vi "GetDesiredHeading.vi"(10 "QueueRef":T1, 11 "NotifierReff":T2) -> (3 "Desired Heading":dbl)   [LabVIEW 2013]
doc: "This VI takes the waypoint queue, looks at the first element, and makes the desired heading the angle to that point.\n\nIn the future, we could make the boat ignore desired headins in irons or pointed at obstacles. That code should go in here.\n\nEric Schneider, March 2014"
uses:
  Data/TypeDefs/Notifiers.ctl
  Data/TypeDefs/UTM Location.ctl
  Data/TypeDefs/Sail Set Suggestions.ctl
  Data/TypeDefs/Rudder Set Suggestions.ctl
  Data/TypeDefs/OverrideInformation.ctl
  Data/TypeDefs/OverrideMode.ctl
  Data/TypeDefs/Queues.ctl
  Classes/Waypoint/Waypoint.lvclass
  Classes/Missions/GenericMission/GenericMission.lvclass
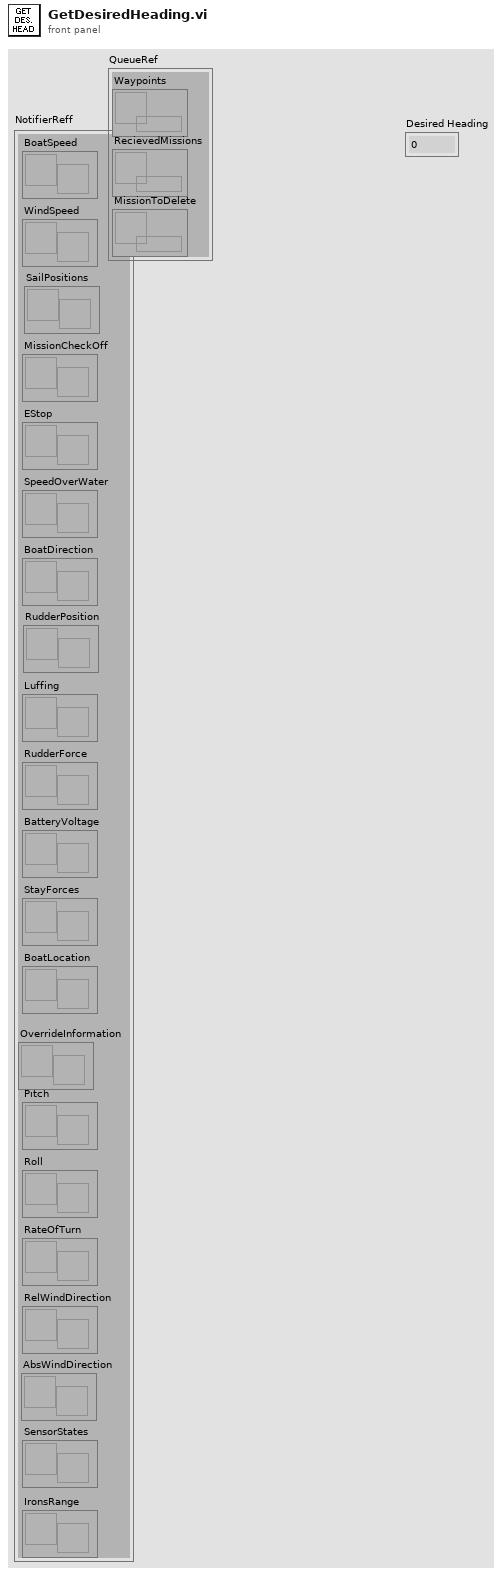
[diagram p1: front panel]
types:
  T1 = typedef "Queues.ctl" = cluster{"Waypoints":refnum<queue>, "RecievedMissions":refnum<queue>, "MissionToDelete":refnum<queue>}
  T2 = typedef "Notifiers.ctl" = cluster{"BoatSpeed":refnum<notifier>, "WindSpeed":refnum<notifier>, "MissionCheckOff":refnum<notifier>, "EStop":refnum<notifier>, "SpeedOverWater":refnum<notifier>, "BoatDirection":refnum<notifier>, "Luffing":refnum<notifier>, "RudderForce":refnum<notifier>, "BatteryVoltage":refnum<notifier>, "StayForces":refnum<notifier>, "BoatLocation":refnum<notifier>, "Pitch":refnum<notifier>, "Roll":refnum<notifier>, "RateOfTurn":refnum<notifier>, "RelWindDirection":refnum<notifier>, "SailPositions":refnum<notifier>, "RudderPosition":refnum<notifier>, "SensorStates":refnum<notifier>, "IronsRange":refnum<notifier>, "AbsWindDirection":refnum<notifier>, "OverrideInformation":refnum<notifier>}
  T3 = typedef "UTM Location.ctl" = cluster{"UTM Zone":dbl, "Hemisphere":enum16{"North", "South"}, "East":dbl, "North":dbl}
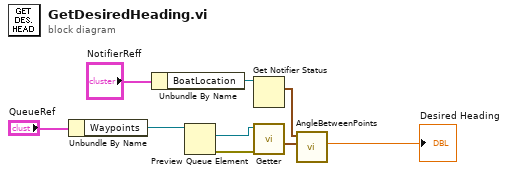
[diagram p0: block diagram]
diagram:
  n1 = Unbundle By Name("QueueRef") -> ("Waypoints"=w4:refnum<queue>)
  n2 = Unbundle By Name("NotifierReff") -> ("BoatLocation"=w6:refnum<notifier>)
  n3 = Preview Queue Element(queue=w4) -> (element=w3:refnum<class "Waypoint.lvclass">, error out=w2:errorcluster)  [unwired: 2 in, 2 out]
  n4 = Get Notifier Status(notifier=w6) -> (current notification=w8:T3)  [unwired: 1 in, 4 out]
  n5 = call "Getter.vi"("Error In"=w2, "Waypoint In"=w3) -> ("Coords"=w9:T3)  [unwired: 5 in, 4 out]
  n6 = call "AngleBetweenPoints.vi"("Point 2"=w9, "Point 1"=w8) -> ("Angle"=→"Desired Heading":dbl)  [unwired: 9 in]
